vi "SRV_Check and Set VI Inputs.vi"(6 "Callback Identifier":string, 8 "error in (no error)":errorcluster, 9 "Optional Controls (none)":cluster{"Name":string, "Value":variant}[](array[cluster]), 10 "Required Controls":cluster{"Name":string, "Value":variant}[](array[cluster]), 11 "VI Refnum In":refnum<vi>) -> (0 "error out":errorcluster, 3 "VI Refnum Out":refnum<vi>)   [LabVIEW 2009]
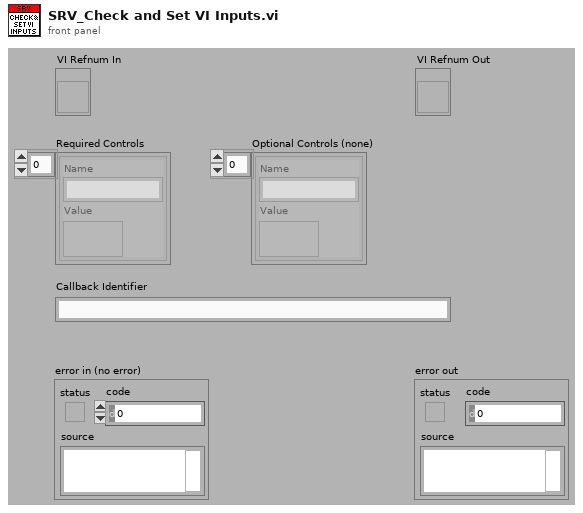
[diagram p1: front panel]
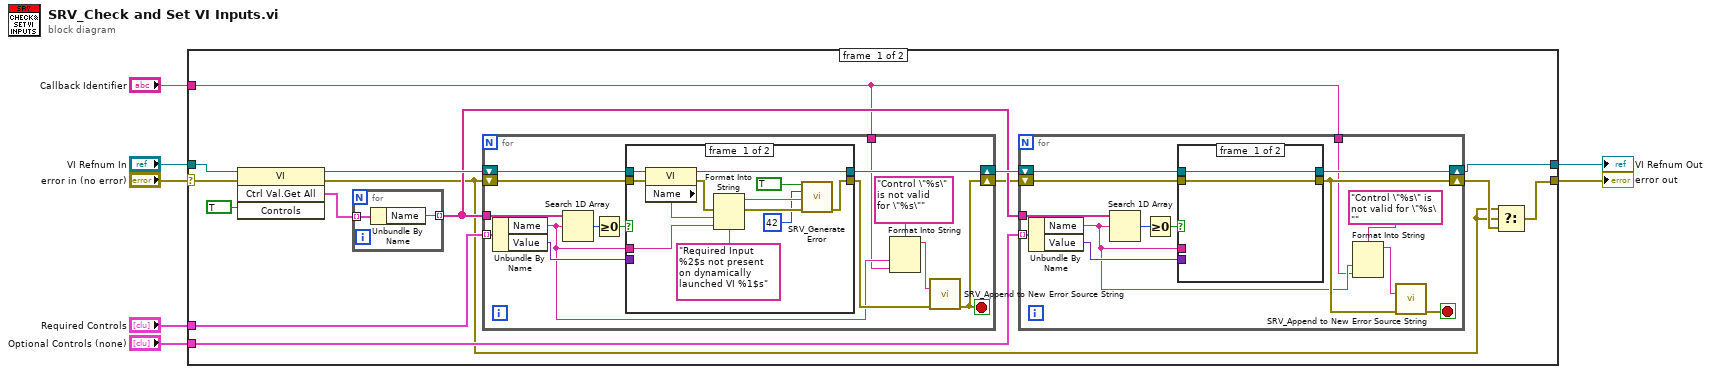
[diagram p0: block diagram]
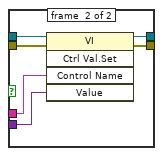
[diagram p2: hidden frame]
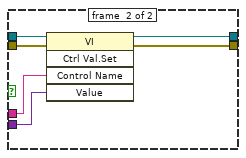
[diagram p3: hidden frame]
diagram:
  n1 = case shown="No Error" "error in (no error)" {
    selector: "error in (no error)" -> [w17 w80]
    tunnel: "VI Refnum In" -> [w21 w79]
    tunnel: "Required Controls" -> [w19 _]
    tunnel: "Optional Controls (none)" -> [w14 _]
    tunnel: [w13 w79] -> w4
    tunnel: [w11 w80] -> w3
    tunnel: "Callback Identifier" -> [w8 _]
    frame #0 {
      n2 = invoke class="VI" method="Ctrl Val.Get All"(reference=w21, error in=w17, "Controls"=TRUE) -> (reference out=w18:refnum<vi>, error out=w9:errorcluster, "Get All Control Values Variant"=w20:cluster{"Name":string, "Variant Data":variant}[])  [unwired: 1 in, 1 out]
      n3 = for {
        tunnel: w20 -> [w78] mode=indexing
        tunnel: [w77] -> w15 mode=indexing
        n4 = Unbundle By Name(w78) -> ("Name"=w77:string)
      }
      n5 = for {
        tunnel: w15 -> [w58]
        tunnel: w19 -> [w57] mode=indexing
        shift-right: [w51] -> w16
        shift-left: w18 -> [w56]
        shift-right: [w47] -> w10
        shift-left: w9 -> [w53]
        tunnel: w8 -> [w45]
        stop <- w47 stop-if-true
        n6 = Unbundle By Name(w57) -> ("Name"=w46:string, "Value"=w52:variant)
        n7 = Search 1D Array(1D array=w58, element=w46) -> (index of element=w55:i32)  [unwired: 1 in]
        n8 = Greater Or Equal To 0?(x=w55) -> (x >= 0?=w54:bool)
        n9 = case shown="True" w54 {
          tunnel: w56 -> [w70 w76]
          tunnel: w53 -> [w69 w75]
          tunnel: w46 -> [w64 w74]
          tunnel: w52 -> [_ w73]
          tunnel: [w66 w71] -> w51
          tunnel: [w59 w72] -> w48
          frame #0 {
            n10 = property class="VI"(reference=w70, error in=w69) -> (reference out=w66:refnum<vi>, error out=w67:errorcluster, "Name"=w65:string)
            n11 = Format Into String(format string="Required Input %2$s not present on dynamically launched VI %1$s", error in=w67, w65, w64) -> (resulting string=w62:string, error out=w63:errorcluster)  [unwired: 1 in]
            n12 = call "SRV_Generate Error.vi"("status (T)"=TRUE ("status (F)"), "code (42: generic error)"=42 ("code (0: no error)"), "Message"=w62, "error in (no error)"=w63) -> ("error out"=w59:errorcluster)  [unwired: 11 in]
          }
          frame #1 {
            n13 = invoke class="VI" method="Ctrl Val.Set"(reference=w76, error in=w75, "Control Name"=w74, "Value"=w73) -> (reference out=w71:refnum<vi>, error out=w72:errorcluster)  [unwired: 1 in, 3 out]
          }
        }
        n14 = Format Into String(format string="Control \"%s\" is not valid for \"%s\"", w46, w45) -> (resulting string=w49:string)  [unwired: 2 in, 1 out]
        n15 = call "SRV_Append to New Error Source String.vi"("Message String to append"=w49, "Error In (no error)"=w48) -> ("error out"=w47:errorcluster)  [unwired: 13 in]
      }
      n16 = for {
        tunnel: w15 -> [w36]
        tunnel: w14 -> [w35] mode=indexing
        shift-right: [w29] -> w13
        shift-left: w16 -> [w34]
        shift-right: [w27] -> w12
        shift-left: w10 -> [w31]
        tunnel: w8 -> [w25]
        stop <- w28 stop-if-true
        n17 = Unbundle By Name(w35) -> ("Name"=w26:string, "Value"=w30:variant)
        n18 = Search 1D Array(1D array=w36, element=w26) -> (index of element=w33:i32)  [unwired: 1 in]
        n19 = Greater Or Equal To 0?(x=w33) -> (x >= 0?=w32:bool)
        n20 = case shown="True" w32 {
          tunnel: w34 -> [w37 w44]
          tunnel: w31 -> [w38 w43]
          tunnel: w26 -> [_ w42]
          tunnel: w30 -> [_ w41]
          tunnel: [w37 w39] -> w29
          tunnel: [w38 w40] -> w27
          frame #0 {
          }
          frame #1 {
            n21 = invoke class="VI" method="Ctrl Val.Set"(reference=w44, error in=w43, "Control Name"=w42, "Value"=w41) -> (reference out=w39:refnum<vi>, error out=w40:errorcluster)  [unwired: 1 in, 3 out]
          }
        }
        n22 = Format Into String(format string="Control \"%s\" is not valid for \"%s\"", w26, w25) -> (resulting string=w23:string)  [unwired: 2 in, 1 out]
        n23 = call "SRV_Append to New Error Source String.vi"("Message String to append"=w23, "Error In (no error)"=w27) -> ("error out"=w28:errorcluster)  [unwired: 13 in]
      }
      n24 = Select(t=w9, s=w9, f=w12) -> (s? t:f=w11:errorcluster)
    }
    frame #1 {
    }
  }
  "VI Refnum Out" <- w4
  "error out" <- w3
